vi "List Packages in Feed.vi"(8 "error in":errorcluster, 11 "feed folderpath in":path) -> (0 "error out":errorcluster, 1 "package names and versions":string[][](array[string]), 2 "package relative filepaths":path[](array[path]), 3 "feed folderpath out":path)   [LabVIEW 2014, in "NIPM_API.lvlib"]
doc: "Retuns a list of all the packages in the specified feed\n\nINPUT(s)\n<B>Feed folderpath</B>: Specifies the folder containing the feed\n\nOUTPUT(s)\n<B>Feed folderpath out</B>: Outputs the specified feed folderpath\n\n<B>Package relative filepaths</B>: Outputs 1D array that lists the feed's package filepaths (.nipkg) relative to the location of the feed manifest files (Packages, Packages.gz, Packages.stamps)\n\n<B>Package names and versions</B>: Outputs a 2D string array listing the package names and versions in the feed"
uses:
  NIPM_API.lvlib
  <vilib>/Utility/file.llb/Read From Spreadsheet File (string).vi
panel:
  # "Array\n\npackage name     version      visible?"
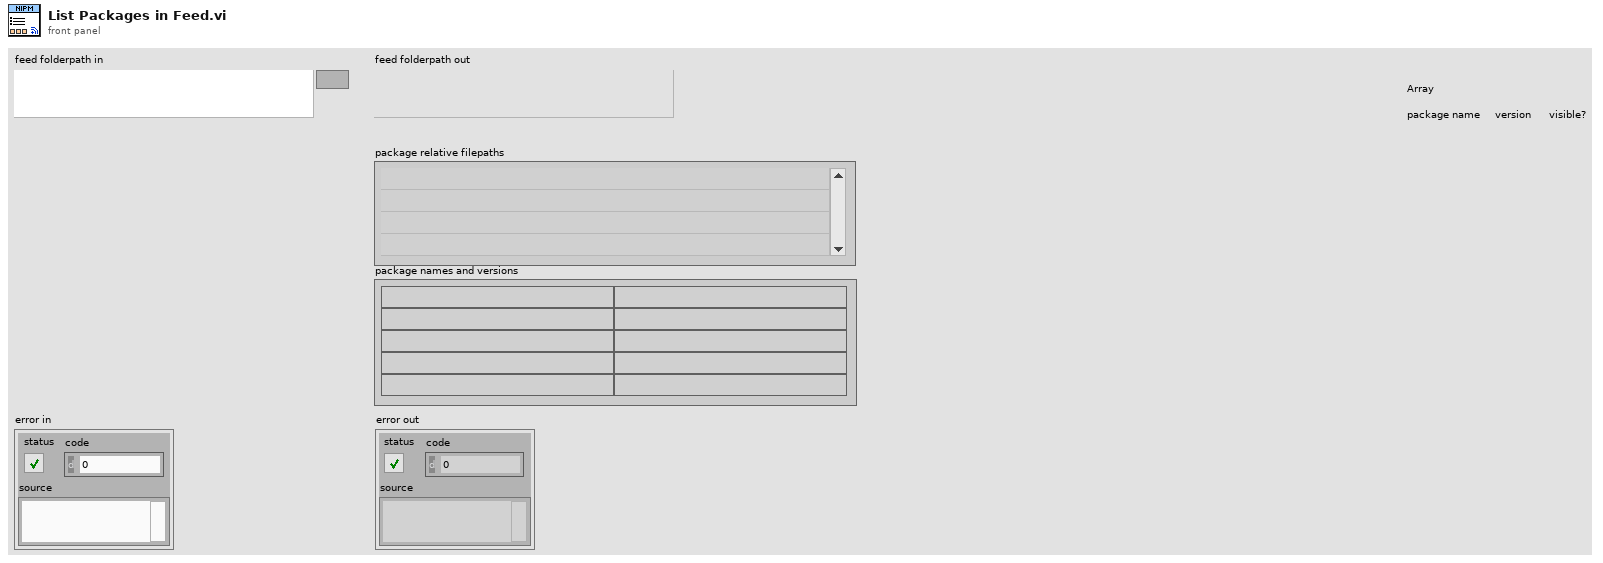
[diagram p1: front panel]
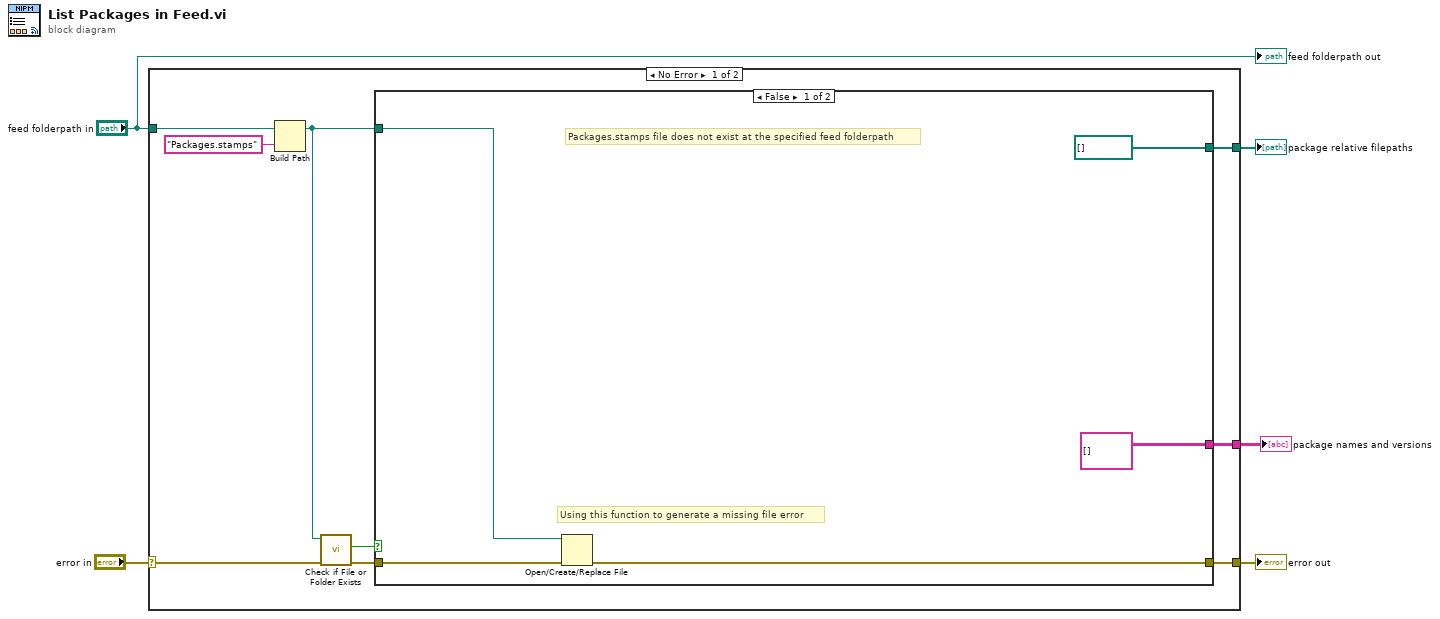
[diagram p0: block diagram]
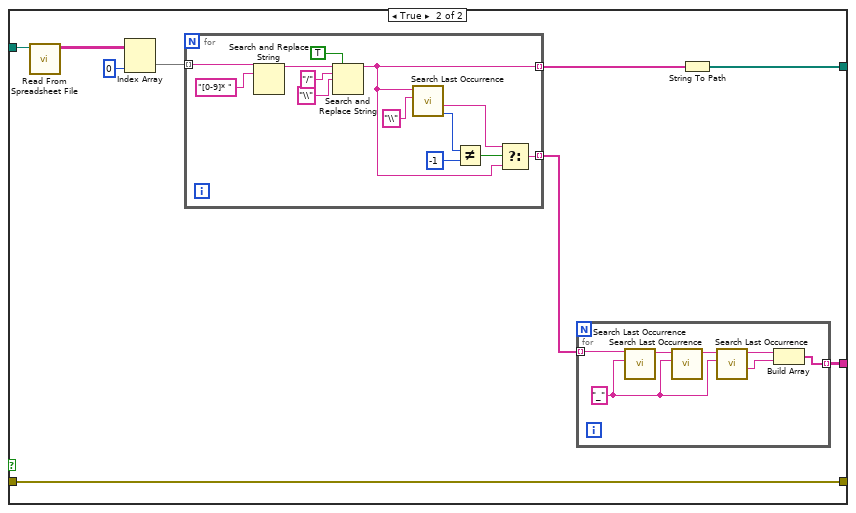
[diagram p2: hidden frame]
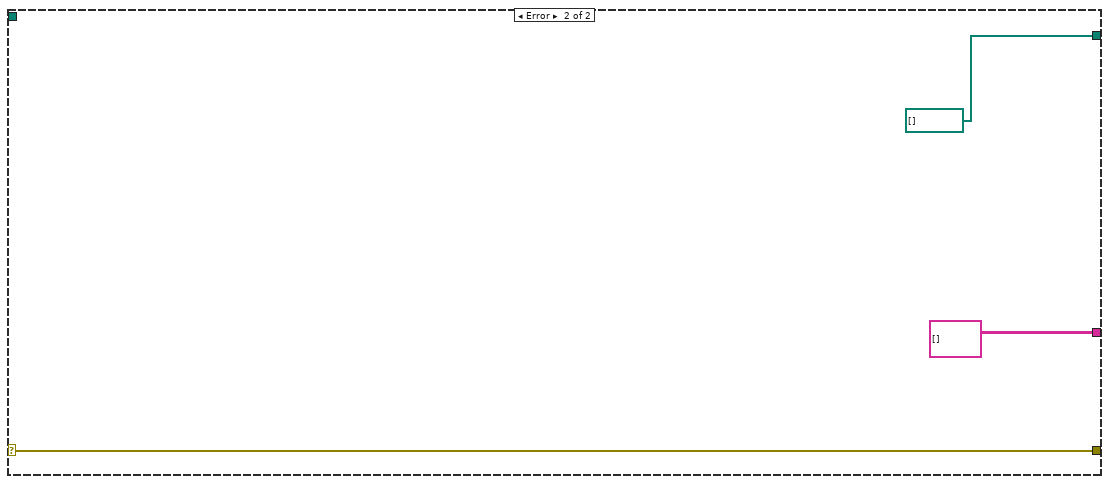
[diagram p3: hidden frame]
diagram:
  n1 = case shown="No Error" "error in" {
    selector: "error in" -> [w10 w51]
    tunnel: "feed folderpath in" -> [w14 _]
    tunnel: [w11 path[] []] -> w5
    tunnel: [w13 string[][] []] -> w4
    tunnel: [w6 w51] -> w2
    frame No Error {
      n2 = Build Path(base path=w14, name or relative path="Packages.stamps") -> (appended path=w9:path)
      n3 = call <vilib>:"Check if File or Folder Exists.vi"("error in (no error)"=w10, "path"=w9) -> ("error out"=w7:errorcluster, "file or folder exists?"=w8:bool)  [unwired: 7 in, 1 out]
      n4 = case shown="False" w8 {
        tunnel: [string[][] [] w25] -> w13
        tunnel: [path[] [] w22] -> w11
        tunnel: w9 -> [w17 w21]
        tunnel: w7 -> [w16 w20]
        tunnel: [w15 w20] -> w6
        frame False {
          # "Packages.stamps file does not exist at the specified feed folderpath"
          # "Using this function to generate a missing file error"
          n5 = Open/Create/Replace File(file path (use dialog)=w17, error in=w16) -> (error out=w15:errorcluster)  [unwired: 4 in, 2 out]
        }
        frame True {
          n6 = call-poly <vilib>:"Read From Spreadsheet File.vi"("file path (dialog if empty)"=w21) -> ("all rows"=w24:string[][])  [unwired: 6 in, 4 out]
          n7 = Index Array(array=w24, index (col)=0 ("disabled index (col)")) -> (element=w27:string[])  [unwired: 1 in]
          n8 = for {
            tunnel: w27 -> [w48] mode=indexing
            tunnel: [w44] -> w26 mode=indexing
            tunnel: [w36] -> w23 mode=indexing
            n9 = Search and Replace String(input string=w48, search string="[0-9]* ") -> (result string=w37:string)  [unwired: 6 in, 3 out]
            n10 = Search and Replace String(replace all?=TRUE ("replace all? (F)"), input string=w37, search string="/", replace string="\\" ("replace string (\"\")")) -> (result string=w36:string)  [unwired: 4 in, 3 out]
            n11 = call "Search Last Occurrence.vi"("search string/char (-)"="\\", "string"=w36) -> ("offset of match"=w42:i32, "rest of string"=w41:string)  [unwired: 6 in, 2 out]
            n12 = Not Equal?(x=w42, y=-1) -> (x != y?=w45:bool)
            n13 = Select(t=w41, s=w45, f=w36) -> (s? t:f=w44:string)
          }
          n14 = for {
            tunnel: w26 -> [w35] mode=indexing
            tunnel: [w29] -> w25 mode=indexing
            w32 = "_" ("search string/char (-)")
            n15 = call "Search Last Occurrence.vi"("search string/char (-)"=w32, "string"=w35) -> ("substring before match"=w34:string)  [unwired: 6 in, 3 out]
            n16 = call "Search Last Occurrence.vi"("search string/char (-)"=w32, "string"=w34) -> ("substring before match"=w33:string)  [unwired: 6 in, 3 out]
            n17 = call "Search Last Occurrence.vi"("search string/char (-)"=w32, "string"=w33) -> ("rest of string"=w30:string, "substring before match"=w31:string)  [unwired: 6 in, 2 out]
            n18 = Build Array(w31, w30) -> (w29:string[])
          }
          n19 = String To Path(string=w23) -> (path=w22:path[])
        }
      }
    }
    frame Error {
    }
  }
  "package relative filepaths" <- w5
  "error out" <- w2
  "package names and versions" <- w4
  "feed folderpath out" <- "feed folderpath in"
